vi "Shut Down Device.vi"(8 "error in (no error)":errorcluster, 11 "Andor Camera in":refnum<class "Andor Camera.lvclass">) -> (0 "error out":errorcluster, 3 "Andor Camera out":refnum<class "Andor Camera.lvclass">)   [LabVIEW 2018, in "Andor Camera.lvlib" / "Andor Camera.lvclass"]
uses:
  Andor Camera.lvclass
  Camera/Camera.lvclass
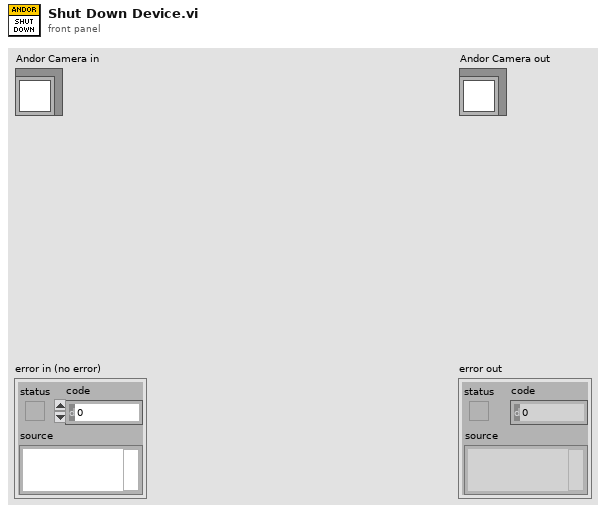
[diagram p1: front panel]
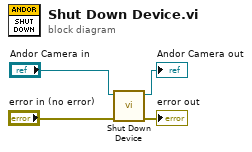
[diagram p0: block diagram]
diagram:
  n1 = call-parent "Shut Down Device.vi"("error in (no error)"="error in (no error)", "Device in"="Andor Camera in") -> ("error out"=→"error out":errorcluster, "Device out"=→"Andor Camera out":refnum<class "Andor Camera.lvclass">)  [unwired: 8 in]
